vi "S7 Close.vi"(8 "Error In":errorcluster, 11 "TCP In":refnum<k5>) -> (0 "error out":errorcluster caption="Error Out")   [LabVIEW 2020]
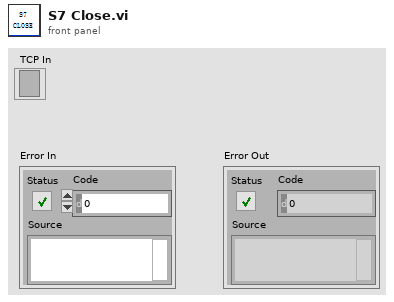
[diagram p1: front panel]
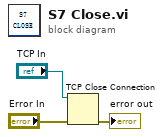
[diagram p0: block diagram]
diagram:
  n1 = TCP Close Connection(connection ID="TCP In", error in (no error)="Error In") -> (error out=→"error out":errorcluster)  [unwired: 1 in, 1 out]
